vi "acidFlush.vi"() -> ()   [LabVIEW 2010]
panel:
  out "VISA resource out":refnum<visa-resource-name>="ASRL2::INSTR"
  in  "Action 2":u8(ring) items=["TurnON_1"=8, "TurnON_PUMP"=9, "TurnON_3"=10, "TurnON_4"=11, "TurnOFF_1"=0, "TurnOFF_PUMP"=1, "TurnOFF_3"=2, "TurnOFF_4"=3, "OpenAll"=30, "CloseAllRelay"=29]
  in  "VISA resource name":refnum<visa-resource-name>="ASRL2::INSTR"
  in  "error in":errorcluster
  out "error out":errorcluster
  in  "Action":u8(ring) items=["TurnON_1"=8, "TurnON_PUMP"=9, "TurnON_3"=10, "TurnON_4"=11, "TurnOFF_1"=0, "TurnOFF_PUMP"=1, "TurnOFF_3"=2, "TurnOFF_4"=3, "OpenAll"=30, "CloseAllRelay"=29]
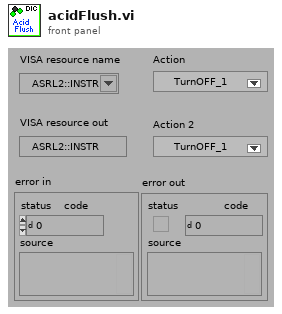
[diagram p1: front panel]
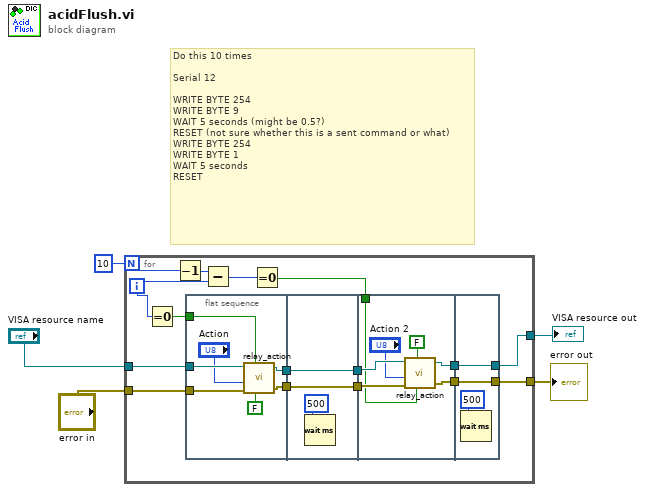
[diagram p0: block diagram]
diagram:
  # "Do this 10 times\n\nSerial 12\n\nWRITE BYTE 254\nWRITE BYTE 9\nWAIT 5 seconds (might be 0.5?)\nRESET (not sure whether this is a sent command or what)\nWRITE BYTE 254\nWRITE BYTE 1\nWAIT 5 seconds\nRESET"
  n1 = for {
    N: 10 -> [w14]
    tunnel: "VISA resource name" -> [w20]
    tunnel: "error in" -> [w19]
    tunnel: [w7] -> w2
    tunnel: [w6] -> w1
    i -> [w12]
    n2 = Equal To 0?(x=w12) -> (x = 0?=w21:bool)
    n3 = Decrement(x=w14) -> (x-1=w13:i32)
    n4 = flat-sequence {
      tunnel: w21 -> [w28]
      tunnel: w20 -> [w27]
      tunnel: w19 -> [w26]
      tunnel: [w24] -> w17
      tunnel: [w23] -> w15
      tunnel: [w30] -> w18
      tunnel: w17 -> [w30]
      tunnel: [w29] -> w16
      tunnel: w15 -> [w29]
      tunnel: w18 -> [w36]
      tunnel: w16 -> [w38]
      tunnel: w10 -> [w34]
      tunnel: [w33] -> w9
      tunnel: [w32] -> w8
      tunnel: [w40] -> w7
      tunnel: [w41] -> w6
      tunnel: w9 -> [w41]
      tunnel: w8 -> [w40]
      frame #0 {
        n5 = call "relay_action.vi"("VISA resource name"=w27, "init?"=w28, "Action"="Action", "Quit?"=FALSE, "error in"=w26) -> ("VISA resource name 2"=w24:refnum<visa-resource-name>, "error out"=w23:errorcluster)  [unwired: 2 in]
      }
      frame #1 {
        n6 = Wait (ms)(milliseconds to wait=500) -> ()  [unwired: 1 out]
      }
      frame #2 {
        n7 = call "relay_action.vi"("VISA resource name"=w36, "init?"=FALSE, "Action"="Action 2", "Quit?"=w34, "error in"=w38) -> ("VISA resource name 2"=w33:refnum<visa-resource-name>, "error out"=w32:errorcluster)  [unwired: 2 in]
      }
      frame #3 {
        n8 = Wait (ms)(milliseconds to wait=500) -> ()  [unwired: 1 out]
      }
    }
    n9 = Subtract(x=w13, y=w12) -> (x-y=w11:i32)
    n10 = Equal To 0?(x=w11) -> (x = 0?=w10:bool)
  }
  "error out" <- w2
  "VISA resource out" <- w1
